vi "Thermal Chamber Controller with DUT.vi"() -> ()   [LabVIEW 2020]
uses:
  Thermal Chamber Controller/Thermal Chamber Controller.lvclass
  C:/Program Files (x86)/National Instruments/LabVIEW 2020/vi.lib/Asteme/Triarc Framework/Process/Process.lvclass
  C:/Program Files (x86)/National Instruments/LabVIEW 2020/vi.lib/Asteme/Triarc Framework/View/View.lvclass
  Thermal Chamber Controller/Private/Heater State.ctl
  Device Under Test/Device Under Test.lvclass
  <vilib>/Asteme/Triarc Framework/Process/Process.lvclass/Process.ctl
  <vilib>/Asteme/Triarc Framework/View/View.lvclass/View.ctl
  <vilib>/Asteme/Triarc Framework/Process/Protected/Messaging/Enqueue Message.vi
  <vilib>/Asteme/Triarc Framework/View/Public/Get View VI Reference.vi
  <vilib>/Asteme/Triarc Framework/Process/Public/Lifecycle/Get Lifecycle State.vi
  <vilib>/Asteme/Triarc Framework/Process/Private/SubVIs/Wait for finish.vi
  <vilib>/Asteme/Triarc Framework/Process/Private/SubVIs/Set Lifecycle State.vi
  <vilib>/Asteme/Triarc Framework/Process/Protected/Messaging/Request Message.vi
  <vilib>/Utility/error.llb/Clear Errors.vi
  <vilib>/Asteme/Triarc Framework/Process/Private/SubVIs/Enqueue Request Message.vi
  <vilib>/Asteme/Triarc Framework/View/View.lvclass
  <vilib>/Utility/error.llb/Error Cluster From Error Code.vi
  <vilib>/Asteme/Triarc Framework/Process/Private/SubVIs/Wait for Response Message.vi
  <vilib>/Asteme/Triarc Framework/Process/Process.lvclass
panel:
  out "Self Test Result":bool
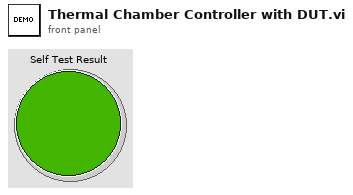
[diagram p1: front panel]
types:
  T1 = typedef "Thermal Chamber Controller.lvclass/Heater State.ctl" = enum16{"Heater Disabled", "Heater Enabled"}
  T2 = typedef "Thermal Chamber Controller.lvclass/Chamber State.ctl" = cluster{"Actual Temperature":dbl, "Temperature Set Point":dbl, "Temperature Ramp Rate":dbl, "Heater State":T1}
  T3 = typedef "Device Under Test.lvclass/Self Test Reply Payload.ctl" = cluster{"Result":bool, "Self Test Error":errorcluster}
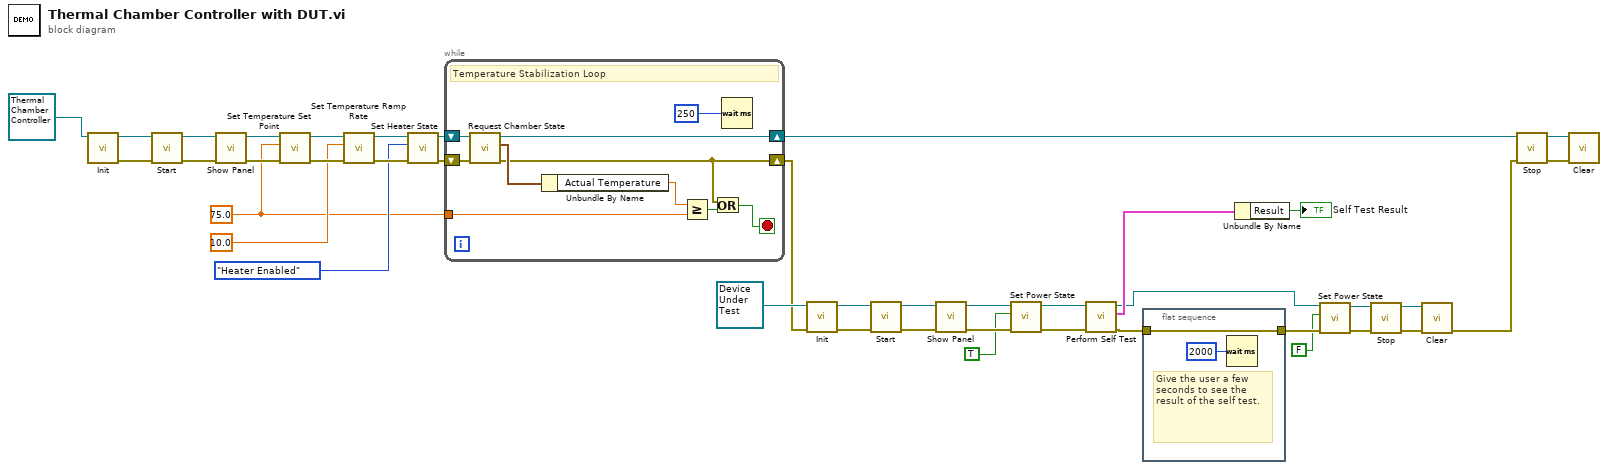
[diagram p0: block diagram]
diagram:
  w23 = 75.0 ("Temperature Set Point")
  n1 = call-dynamic "Init.vi"("View In"=refnum<class "Thermal Chamber Controller.lvclass"> refnum ("Thermal Chamber Controller.lvclass")) -> ("error out"=w40:errorcluster, "View Out"=w41:refnum<class "Thermal Chamber Controller.lvclass">)  [unwired: 9 in]
  n2 = call <vilib>:"Start.vi"("error in (no error)"=w40, "Process In"=w41) -> ("error out"=w39:errorcluster, "Process Out"=w34:refnum<class "Thermal Chamber Controller.lvclass">)  [unwired: 8 in]
  n3 = call <vilib>:"Show Panel.vi"("error in (no error)"=w39, "View In"=w34) -> ("error out"=w35:errorcluster, "View Out"=w32:refnum<class "Thermal Chamber Controller.lvclass">)  [unwired: 8 in]
  n4 = call "Set Temperature Set Point.vi"("error in (no error)"=w35, "Temperature Set Point"=w23, "Thermal Chamber Controller In"=w32) -> ("error out"=w33:errorcluster, "Thermal Chamber Controller Out"=w30:refnum<class "Thermal Chamber Controller.lvclass">)  [unwired: 7 in]
  n5 = call "Set Temperature Ramp Rate.vi"("error in (no error)"=w33, "Temperature Ramp Rate [degC/s]"=10.0, "Thermal Chamber Controller In"=w30) -> ("error out"=w31:errorcluster, "Thermal Chamber Controller Out"=w27:refnum<class "Thermal Chamber Controller.lvclass">)  [unwired: 7 in]
  n6 = call "Set Heater State.vi"("error in (no error)"=w31, "Heater State"=Heater_State."Heater Enabled", "Thermal Chamber Controller In"=w27) -> ("error out"=w28:errorcluster, "Thermal Chamber Controller Out"=w25:refnum<class "Thermal Chamber Controller.lvclass">)  [unwired: 7 in]
  n7 = while {
    shift-right: [w46] -> w10
    shift-left: w28 -> [w51]
    shift-right: [w49] -> w24
    shift-left: w25 -> [w50]
    tunnel: w23 -> [w43]
    stop <- w47 stop-if-true
    # "Temperature Stabilization Loop"
    n8 = call "Request Chamber State.vi"("error in (no error)"=w51, "Thermal Chamber Controller In"=w50) -> ("error out"=w46:errorcluster, "Chamber Status Reply Payload"=w48:T2, "Thermal Chamber Controller Out"=w49:refnum<class "Thermal Chamber Controller.lvclass">)  [unwired: 6 in, 1 out]
    n9 = Unbundle By Name(w48) -> ("Actual Temperature"=w44:dbl)
    n10 = Greater Or Equal?(x=w44, y=w43) -> (x >= y?=w42:bool)
    n11 = Or(x=w46, y=w42) -> (x .or. y?=w47:bool)
    n12 = Wait (ms)(milliseconds to wait=u32 250) -> ()  [unwired: 1 out]
  }
  n13 = call-dynamic "Init.vi"("error in (no error)"=w10, "View In"=refnum<class "Device Under Test.lvclass"> refnum ("Device Under Test.lvclass")) -> ("error out"=w20:errorcluster, "View Out"=w19:refnum<class "Device Under Test.lvclass">)  [unwired: 8 in]
  n14 = call <vilib>:"Start.vi"("error in (no error)"=w20, "Process In"=w19) -> ("error out"=w21:errorcluster, "Process Out"=w22:refnum<class "Device Under Test.lvclass">)  [unwired: 8 in]
  n15 = call <vilib>:"Show Panel.vi"("error in (no error)"=w21, "View In"=w22) -> ("error out"=w16:errorcluster, "View Out"=w17:refnum<class "Device Under Test.lvclass">)  [unwired: 8 in]
  n16 = call "Set Power State.vi"("error in (no error)"=w16, "Power State"=TRUE, "Device Under Test In"=w17) -> ("error out"=w14:errorcluster, "Device Under Test Out"=w15:refnum<class "Device Under Test.lvclass">)  [unwired: 7 in]
  n17 = call "Perform Self Test.vi"("error in (no error)"=w14, "Device Under Test In"=w15) -> ("error out"=w12:errorcluster, "data"=w8:T3, "Device Under Test Out"=w3:refnum<class "Device Under Test.lvclass">)  [unwired: 6 in, 1 out]
  n18 = flat-sequence {
    tunnel: w12 -> [w53]
    tunnel: [w53] -> w11
    frame #0 {
      # "Give the user a few seconds to see the result of the self test."
      n19 = Wait (ms)(milliseconds to wait=u32 2000) -> ()  [unwired: 1 out]
    }
  }
  n20 = Unbundle By Name(w8) -> ("Result"=→"Self Test Result":bool)
  n21 = call "Set Power State.vi"("error in (no error)"=w11, "Power State"=FALSE, "Device Under Test In"=w3) -> ("error out"=w2:errorcluster, "Device Under Test Out"=w4:refnum<class "Device Under Test.lvclass">)  [unwired: 7 in]
  n22 = call <vilib>:"Stop.vi"("error in (no error)"=w2, "Process In"=w4) -> ("error out"=w6:errorcluster, "Process Out"=w5:refnum<class "Device Under Test.lvclass">)  [unwired: 7 in, 1 out]
  n23 = call-dynamic "Clear.vi"("error in (no error)"=w6, "View In"=w5) -> ("error out"=w1:errorcluster)  [unwired: 9 in]
  n24 = call <vilib>:"Stop.vi"("error in (no error)"=w1, "Process In"=w24) -> ("error out"=w37:errorcluster, "Process Out"=w38:refnum<class "Thermal Chamber Controller.lvclass">)  [unwired: 7 in, 1 out]
  n25 = call-dynamic "Clear.vi"("error in (no error)"=w37, "View In"=w38) -> ()  [unwired: 9 in, 1 out]
